vi "Caraya Unit Test.vi"   [LabVIEW 2020]
uses:
  Test Symbol.ctl
  <vilib>/addons/_JKI Toolkits/Caraya/classes/Assert/Assert True.vi
  <vilib>/addons/_JKI Toolkits/Caraya/classes/Test/Test.lvclass
  <vilib>/addons/_JKI Toolkits/Caraya/classes/Assert/Assert.lvclass
types:
  T1 = typedef "Test Symbol.ctl" = cluster{"Symbol Name":string, "Symbol Value":string}
  T2 = typedef "Test Results.ctl" = cluster{"Name":string, "Value":string, "Assertion":bool}
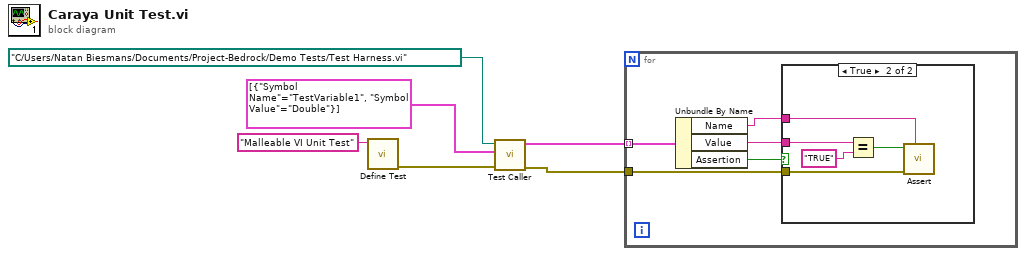
[diagram p0: block diagram]
diagram:
  n1 = call <vilib>:"Define Test.vi"("Label (VI Title)"="Malleable VI Unit Test") -> ("error out"=w5:errorcluster)  [unwired: 9 in, 1 out]
  n2 = call "Test Caller.vi"("error in (no error)"=w5, "Test Symbols"=T1[] [{"Symbol Name"="TestVariable1", "Symbol Value"="Double"}], "Test Harness"=path "C:/Users/Natan Biesmans/Documents/Project-Bedrock/Demo Tests/Test Harness.vi") -> ("error out"=w1:errorcluster, "Results"=w2:T2[])  [unwired: 5 in, 2 out]
  n3 = for {
    tunnel: w2 -> [w11] mode=indexing
    tunnel: w1 -> [w7]
    n4 = Unbundle By Name(w11) -> ("Name"=w8:string, "Value"=w9:string, "Assertion"=w10:bool)
    n5 = case shown="True" w10 {
      tunnel: w9 -> [_ w16]
      tunnel: w8 -> [_ w12]
      tunnel: w7 -> [_ w13]
      frame False {
      }
      frame True {
        n6 = Equal?(x=w16, y="TRUE") -> (x = y?=w14:bool)
        n7 = call-poly <vilib>:"Assert.vi"("Label"=w12, "error in (no error)"=w13, "True?"=w14) -> ()  [unwired: 7 in, 2 out]
      }
    }
  }
